vi "BuildM1RasterSequence.vi"(8 "error in (no error)":errorcluster, 9 "Mode3TestProperties":T2={"Probe Horizontal Polarization"=TRUE, "Probe Vertical Polarization"=FALSE, "Data File Name"="tesrer", "RF In/Out of antenna"=enum."Rx - RF Out", "Raster XY Points"=[{"X mm"=-194.0, "Y mm"=-220.5}, {"X mm"=-47.0, "Y mm"=-220.5}, {"X mm"=100.0, "Y mm"=-220.5}, {"X mm"=247.0, "Y mm"=-220.5}, {"X mm"=-194.0, "Y mm"=-73.5}, {"X mm"=-47.0, "Y mm"=-73.5}, {"X mm"=100.0, "Y mm"=-73.5}, {"X mm"=247.0, "Y mm"=-73.5}, {"X mm"=-194.0, "Y mm"=73.5}, {"X mm"=-47.0, "Y mm"=73.5}, {"X mm"=100.0, "Y mm"=73.5}, {"X mm"=247.0, "Y mm"=73.5}, {"X mm"=-194.0, "Y mm"=220.5}, {"X mm"=-47.0, "Y mm"=220.5}, {"X mm"=100.0, "Y mm"=220.5}, {"X mm"=247.0, "Y mm"=220.5}, {"X mm"=-194.0, "Y mm"=367.5}, {"X mm"=-47.0, "Y mm"=367.5}, {"X mm"=100.0, "Y mm"=367.5}, {"X mm"=247.0, "Y mm"=367.5}]}, 10 "Horizontal T deg":dbl=0.076 format="%#_13g", 11 "Sequence in":refnum<class "Sequence.lvclass">) -> (0 "error out":errorcluster, 2 "PAARD Test Sequence":T4[](array[typedef])=[{"StepType"=enum."Motion", "RF In/Out"=enum."Rx - RF Out", "Module/Raster"=0, "Polarization"=enum."Horizontal", "AO-64 Array"=[], "Position"=[]}, {"StepType"=enum."RasterTest", "RF In/Out"=enum."Tx - RF In", "Module/Raster"=0, "Polarization"=enum."Vertical", "AO-64 Array"=[], "Position"=[]}, {"StepType"=enum."Motion", "RF In/Out"=enum."Rx - RF Out", "Module/Raster"=1, "Polarization"=enum."Horizontal", "AO-64 Array"=[], "Position"=[]}, {"StepType"=enum."RasterTest", "RF In/Out"=enum."Tx - RF In", "Module/Raster"=0, "Polarization"=enum."Vertical", "AO-64 Array"=[], "Position"=[]}, {"StepType"=enum."Motion", "RF In/Out"=enum."Rx - RF Out", "Module/Raster"=2, "Polarization"=enum."Horizontal", "AO-64 Array"=[], "Position"=[]}, {"StepType"=enum."RasterTest", "RF In/Out"=enum."Tx - RF In", "Module/Raster"=0, "Polarization"=enum."Vertical", "AO-64 Array"=[], "Position"=[]}, {"StepType"=enum."Motion", "RF In/Out"=enum."Rx - RF Out", "Module/Raster"=3, "Polarization"=enum."Horizontal", "AO-64 Array"=[], "Position"=[]}, {"StepType"=enum."RasterTest", "RF In/Out"=enum."Tx - RF In", "Module/Raster"=0, "Polarization"=enum."Vertical", "AO-64 Array"=[], "Position"=[]}, {"StepType"=enum."Motion", "RF In/Out"=enum."Rx - RF Out", "Module/Raster"=4, "Polarization"=enum."Horizontal", "AO-64 Array"=[], "Position"=[]}, {"StepType"=enum."RasterTest", "RF In/Out"=enum."Tx - RF In", "Module/Raster"=0, "Polarization"=enum."Vertical", "AO-64 Array"=[], "Position"=[]}, {"StepType"=enum."Motion", "RF In/Out"=enum."Rx - RF Out", "Module/Raster"=5, "Polarization"=enum."Horizontal", "AO-64 Array"=[], "Position"=[]}, {"StepType"=enum."RasterTest", "RF In/Out"=enum."Tx - RF In", "Module/Raster"=0, "Polarization"=enum."Vertical", "AO-64 Array"=[], "Position"=[]}, {"StepType"=enum."Motion", "RF In/Out"=enum."Rx - RF Out", "Module/Raster"=6, "Polarization"=enum."Horizontal", "AO-64 Array"=[], "Position"=[]}, {"StepType"=enum."RasterTest", "RF In/Out"=enum."Tx - RF In", "Module/Raster"=0, "Polarization"=enum."Vertical", "AO-64 Array"=[], "Position"=[]}, {"StepType"=enum."Motion", "RF In/Out"=enum."Rx - RF Out", "Module/Raster"=7, "Polarization"=enum."Horizontal", "AO-64 Array"=[], "Position"=[]}, {"StepType"=enum."RasterTest", "RF In/Out"=enum."Tx - RF In", "Module/Raster"=0, "Polarization"=enum."Vertical", "AO-64 Array"=[], "Position"=[]}, {"StepType"=enum."Motion", "RF In/Out"=enum."Rx - RF Out", "Module/Raster"=8, "Polarization"=enum."Horizontal", "AO-64 Array"=[], "Position"=[]}, {"StepType"=enum."RasterTest", "RF In/Out"=enum."Tx - RF In", "Module/Raster"=0, "Polarization"=enum."Vertical", "AO-64 Array"=[], "Position"=[]}, {"StepType"=enum."Motion", "RF In/Out"=enum."Rx - RF Out", "Module/Raster"=9, "Polarization"=enum."Horizontal", "AO-64 Array"=[], "Position"=[]}, {"StepType"=enum."RasterTest", "RF In/Out"=enum."Tx - RF In", "Module/Raster"=0, "Polarization"=enum."Vertical", "AO-64 Array"=[], "Position"=[]}, {"StepType"=enum."Motion", "RF In/Out"=enum."Rx - RF Out", "Module/Raster"=10, "Polarization"=enum."Horizontal", "AO-64 Array"=[], "Position"=[]}, {"StepType"=enum."RasterTest", "RF In/Out"=enum."Tx - RF In", "Module/Raster"=0, "Polarization"=enum."Vertical", "AO-64 Array"=[], "Position"=[]}, {"StepType"=enum."Motion", "RF In/Out"=enum."Rx - RF Out", "Module/Raster"=11, "Polarization"=enum."Horizontal", "AO-64 Array"=[], "Position"=[]}, {"StepType"=enum."RasterTest", "RF In/Out"=enum."Tx - RF In", "Module/Raster"=0, "Polarization"=enum."Vertical", "AO-64 Array"=[], "Position"=[]}, {"StepType"=enum."Motion", "RF In/Out"=enum."Rx - RF Out", "Module/Raster"=12, "Polarization"=enum."Horizontal", "AO-64 Array"=[], "Position"=[]}, {"StepType"=enum."RasterTest", "RF In/Out"=enum."Tx - RF In", "Module/Raster"=0, "Polarization"=enum."Vertical", "AO-64 Array"=[], "Position"=[]}, {"StepType"=enum."Motion", "RF In/Out"=enum."Rx - RF Out", "Module/Raster"=13, "Polarization"=enum."Horizontal", "AO-64 Array"=[], "Position"=[]}, {"StepType"=enum."RasterTest", "RF In/Out"=enum."Tx - RF In", "Module/Raster"=0, "Polarization"=enum."Vertical", "AO-64 Array"=[], "Position"=[]}, {"StepType"=enum."Motion", "RF In/Out"=enum."Rx - RF Out", "Module/Raster"=14, "Polarization"=enum."Horizontal", "AO-64 Array"=[], "Position"=[]}, {"StepType"=enum."RasterTest", "RF In/Out"=enum."Tx - RF In", "Module/Raster"=0, "Polarization"=enum."Vertical", "AO-64 Array"=[], "Position"=[]}, {"StepType"=enum."Motion", "RF In/Out"=enum."Rx - RF Out", "Module/Raster"=15, "Polarization"=enum."Horizontal", "AO-64 Array"=[], "Position"=[]}, {"StepType"=enum."RasterTest", "RF In/Out"=enum."Tx - RF In", "Module/Raster"=0, "Polarization"=enum."Vertical", "AO-64 Array"=[], "Position"=[]}, {"StepType"=enum."Motion", "RF In/Out"=enum."Rx - RF Out", "Module/Raster"=16, "Polarization"=enum."Horizontal", "AO-64 Array"=[], "Position"=[]}, {"StepType"=enum."RasterTest", "RF In/Out"=enum."Tx - RF In", "Module/Raster"=0, "Polarization"=enum."Vertical", "AO-64 Array"=[], "Position"=[]}, {"StepType"=enum."Motion", "RF In/Out"=enum."Rx - RF Out", "Module/Raster"=17, "Polarization"=enum."Horizontal", "AO-64 Array"=[], "Position"=[]}, {"StepType"=enum."RasterTest", "RF In/Out"=enum."Tx - RF In", "Module/Raster"=0, "Polarization"=enum."Vertical", "AO-64 Array"=[], "Position"=[]}, {"StepType"=enum."Motion", "RF In/Out"=enum."Rx - RF Out", "Module/Raster"=18, "Polarization"=enum."Horizontal", "AO-64 Array"=[], "Position"=[]}, {"StepType"=enum."RasterTest", "RF In/Out"=enum."Tx - RF In", "Module/Raster"=0, "Polarization"=enum."Vertical", "AO-64 Array"=[], "Position"=[]}, {"StepType"=enum."Motion", "RF In/Out"=enum."Rx - RF Out", "Module/Raster"=19, "Polarization"=enum."Horizontal", "AO-64 Array"=[], "Position"=[]}, {"StepType"=enum."RasterTest", "RF In/Out"=enum."Tx - RF In", "Module/Raster"=0, "Polarization"=enum."Vertical", "AO-64 Array"=[], "Position"=[]}, {"StepType"=enum."Finish", "RF In/Out"=enum."Tx - RF In", "Module/Raster"=0, "Polarization"=enum."Vertical", "AO-64 Array"=[], "Position"=[]}], 3 "Sequence out":refnum<class "Sequence.lvclass">, 5 "Axes to Move":T1[](array[typedef]))   [LabVIEW 2018, in "Sequence.lvclass"]
uses:
  Sequence.lvclass
  SequenceSubvis/mWaveTestStep.ctl
  SequenceSubvis/TestStepTypes.ctl
  SequenceSubvis/RF Direction.ctl
  SequenceSubvis/PolarizationSelect.ctl
  APARMainSubvis/VXM Public API/singleAxisMoveDef.ctl
  APARMainSubvis/VXM Public API/mmWaveAxis.ctl
  APARMainSubvis/UI temporary dialogs and VIs/Mode1TestProperties.ctl
  Sequence.lvclass/Sequence.ctl
panel:
  out "# steps":i32=41
  out "length, bytes":i32=1890 format="%.3p"
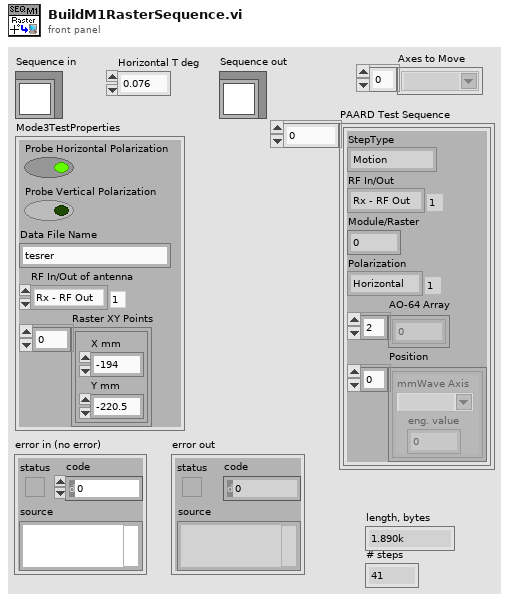
[diagram p1: front panel]
types:
  T1 = typedef "mmWaveAxis.ctl" = string
  T2 = typedef "Mode1TestProperties.ctl" = cluster{"Probe Horizontal Polarization":bool, "Probe Vertical Polarization":bool, "Data File Name":string, "RF In/Out of antenna":T3, "Raster XY Points":cluster{"X mm":dbl, "Y mm":dbl}[]}
  T3 = typedef "RF Direction.ctl" = enum16{"Tx - RF In", "Rx - RF Out"}
  T4 = typedef "mWaveTestStep.ctl" = cluster{"StepType":T5, "RF In/Out":T3, "Module/Raster":i32, "Polarization":T6, "AO-64 Array":dbl[], "Position":T7[]}
  T5 = typedef "TestStepTypes.ctl" = enum16{"MotionFF-M2", "Motion", "SweepTest", "RasterTest", "Finish", "64ModuleCfg"}
  T6 = typedef "PolarizationSelect.ctl" = enum16{"Vertical", "Horizontal"}
  T7 = typedef "singleAxisMoveDef.ctl" = cluster{"mmWave Axis":T1, "eng. value":dbl}
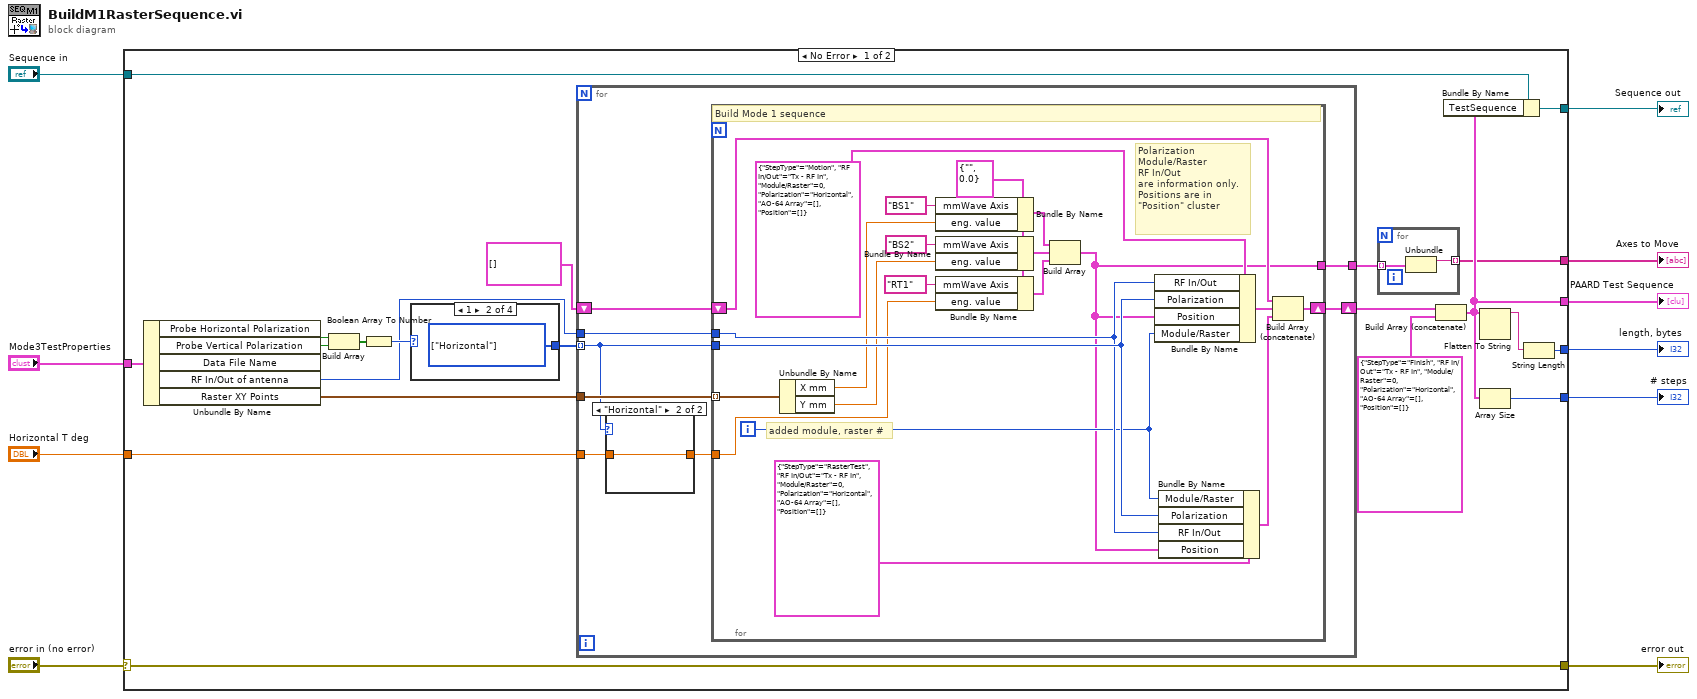
[diagram p0: block diagram]
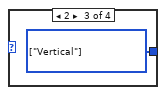
[diagram p3: hidden frame]
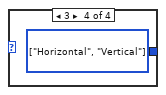
[diagram p4: hidden frame]
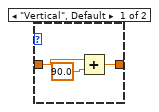
[diagram p5: hidden frame]
diagram:
  n1 = case shown="No Error" "error in (no error)" {
    selector: "error in (no error)" -> [w16 w71]
    tunnel: [w30 _] -> w10
    tunnel: [w13 _] -> w9
    tunnel: [w29 _] -> w8
    tunnel: "Mode3TestProperties" -> [w26 _]
    tunnel: "Horizontal T deg" -> [w19 _]
    tunnel: [w16 w71] -> w5
    tunnel: "Sequence in" -> [w15 w70]
    tunnel: [w14 w70] -> w3
    tunnel: [w11 _] -> w1
    frame No Error {
      n2 = Unbundle By Name(w26) -> ("Probe Horizontal Polarization"=w25:bool, "Probe Vertical Polarization"=w24:bool, "RF In/Out of antenna"=w20:T3, "Raster XY Points"=w18:cluster{"X mm":dbl, "Y mm":dbl}[])  [unwired: 1 out]
      n3 = Build Array(w25, w24) -> (w23:bool[])
      n4 = Boolean Array To Number(Boolean array=w23) -> (number=w22:u32)
      n5 = case shown="1" w22 {
        tunnel: [_ w34 w35 w36] -> w21
        frame 0, Default {
          # "should create an \nerror"
        }
        frame 1 {
          w34 = T6[] [enum."Horizontal"] items=["Vertical", "Horizontal"] ("Polarization(s)")
        }
        frame 2 {
          w35 = T6[] [enum."Vertical"] items=["Vertical", "Horizontal"] ("Polarization(s)")
        }
        frame 3 {
          w36 = T6[] [enum."Horizontal", enum."Vertical"] items=["Vertical", "Horizontal"] ("Polarization(s)")
        }
      }
      n6 = for {
        tunnel: w20 -> [w44]
        tunnel: w18 -> [w43]
        tunnel: w19 -> [w39]
        shift-right: [w42] -> w27
        shift-left: T4[] [] -> [w41]
        tunnel: w21 -> [w40] mode=indexing
        tunnel: [w37] -> w12
        n7 = case shown="\"Horizontal\"" w40 {
          tunnel: [w47 w48] -> w38
          tunnel: w39 -> [w46 w48]
          frame "Vertical", Default {
            n8 = Add(x=w46, y=90.0) -> (x+y=w47:dbl)
          }
          frame "Horizontal" {
          }
        }
        n9 = for {
          tunnel: w44 -> [w62]
          tunnel: w40 -> [w63]
          tunnel: w43 -> [w69] mode=indexing
          shift-right: [w67] -> w42
          shift-left: w41 -> [w66]
          tunnel: w38 -> [w54]
          tunnel: [w49] -> w37
          i -> [w50]
          w60 = T7 {"mmWave Axis"="", "eng. value"=0.0} ("Move")
          # "Polarization\nModule/Raster\nRF In/Out\nare information only.\nPositions are in \n\"Position\" cluster"
          # "added module, raster #"
          # "Build Mode 1 sequence"
          n10 = Unbundle By Name(w69) -> ("X mm"=w56:dbl, "Y mm"=w55:dbl)
          n11 = Bundle By Name(cluster=w60, "mmWave Axis"=T1 "BS1", "eng. value"=w56) -> (w53:T7)
          n12 = Bundle By Name(cluster=w60, "mmWave Axis"=T1 "BS2", "eng. value"=w55) -> (w52:T7)
          n13 = Bundle By Name(cluster=w60, "mmWave Axis"=T1 "RT1", "eng. value"=w54) -> (w51:T7)
          n14 = Build Array(w53, w52, w51) -> (w49:T7[])
          n15 = Bundle By Name(cluster=T4 {"StepType"=enum."Motion", "RF In/Out"=enum."Tx - RF In", "Module/Raster"=0, "Polarization"=enum."Horizontal", "AO-64 Array"=[], "Position"=[]} ("Test"), "RF In/Out"=w62, "Polarization"=w63, "Position"=w49, "Module/Raster"=w50) -> (w68:T4)
          n16 = Bundle By Name(cluster=T4 {"StepType"=enum."RasterTest", "RF In/Out"=enum."Tx - RF In", "Module/Raster"=0, "Polarization"=enum."Horizontal", "AO-64 Array"=[], "Position"=[]} ("Test"), "Module/Raster"=w50, "Polarization"=w63, "RF In/Out"=w62, "Position"=w49) -> (w64:T4)
          n17 = Build Array (concatenate)(w66, w68, w64) -> (w67:T4[])
        }
      }
      n18 = for {
        tunnel: w12 -> [w33] mode=indexing
        tunnel: [w32] -> w11 mode=indexing
        n19 = Unbundle(w33) -> ("mmWave Axis"=w32:T1)  [unwired: 1 out]
      }
      n20 = Build Array (concatenate)(w27, T4 {"StepType"=enum."Finish", "RF In/Out"=enum."Tx - RF In", "Module/Raster"=0, "Polarization"=enum."Horizontal", "AO-64 Array"=[], "Position"=[]} ("Test")) -> (w13:T4[])
      n21 = Bundle By Name(cluster=w15, "TestSequence"=w13) -> (w14:refnum<class "Sequence.lvclass">)
      n22 = Flatten To String(anything=w13) -> (data string=w31:string)  [unwired: 3 in, 2 out]
      n23 = Array Size(array=w13) -> (size(s)=w29:i32)
      n24 = String Length(string=w31) -> (length=w30:i32)
    }
    frame Error {
    }
  }
  "error out" <- w5
  "Sequence out" <- w3
  "PAARD Test Sequence" <- w9
  "length, bytes" <- w10
  "# steps" <- w8
  "Axes to Move" <- w1
